vi "Can_Be_Package_Top_Level.vi"(8 "error in (no error)":errorcluster, 9 "AB_Source in":refnum<class "AB_Source.lvclass">, 11 "Build in":refnum<class "AB_Targetfile.lvclass">) -> (0 "error out":errorcluster, 2 "topLevel":bool, 3 "Build out":refnum<class "AB_Targetfile.lvclass">)   [LabVIEW 2020, in "AB_Targetfile.lvclass"]
uses:
  <vilib>/AppBuilder/AB_Classes/TargetFile/AB_Targetfile.lvclass
  <vilib>/AppBuilder/AB_Classes/Source/AB_Source.lvclass
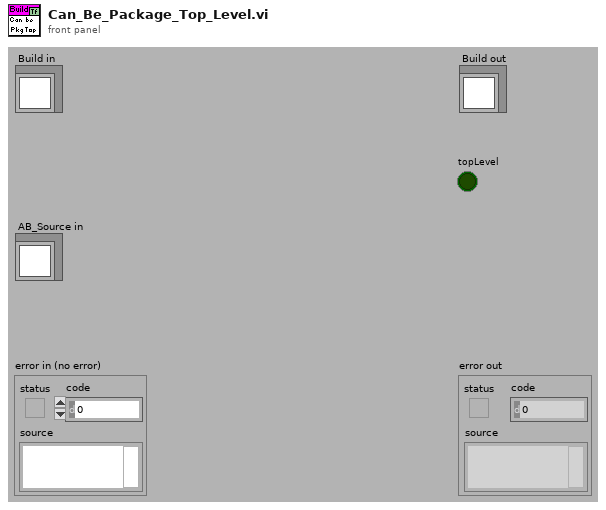
[diagram p1: front panel]
types:
  T1 = typedef "AB_Source.ctl" = cluster{"path":path, "itemID":string, "parentIndex":i32, "sourceInclusion":T2, "destinationIndex":i32, "properties":T3[], "newName":string, "lvfile":bool, "valid":bool, "eng_inBuild":bool, "eng_isNonVILink":bool, "Amalgamation":bool, "Amalgamation Piece":bool, "eng_delimitedName":string, "preventRename":bool}
  T2 = typedef "AB_Source_Inclusion.ctl" = enum16{"IncludeIfReferenced", "Include", "Exclude", "TopLevel"}
  T3 = typedef "AB_Source_Properties.ctl" = cluster{"sourcePropertyType":T4, "value":variant}
  T4 = typedef "AB_Source_Property_Type.ctl" = enum16{"Remove block diagram", "Remove front panel", "Password", "Window has title bar", "Show menu bar", "Show vertical scroll bar", "Show horizontal scroll bar", "Show toolbar", "Show Abort button", "Show fp when called", "Window behavior", "Allow user to close window", "Window run-time position", "Run when opened", "Allow debugging", "Auto error handling", "Generate guard code", "Use stack variables", "Expression folding", "Integer only", "Inline subVI"}
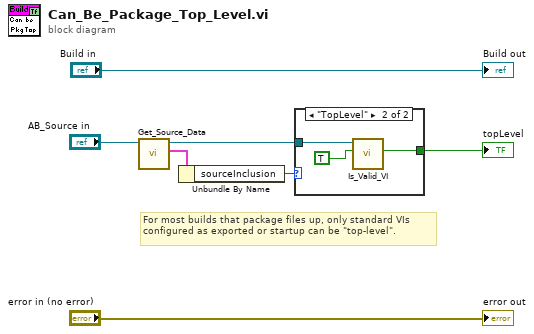
[diagram p0: block diagram]
diagram:
  # "For most builds that package files up, only standard VIs configured as exported or startup can be \"top-level\"."
  n1 = call <vilib>:"Get_Source_Data.vi"("Class in"="AB_Source in") -> ("data"=w5:T1, "Class out"=w3:refnum<class "AB_Source.lvclass">)  [unwired: 1 in, 8 out]
  n2 = Unbundle By Name(w5) -> ("sourceInclusion"=w2:T2)
  n3 = case shown="\"TopLevel\"" w2 {
    tunnel: w3 -> [_ w9]
    tunnel: [_ w8] -> w1
    frame Default {
    }
    frame "TopLevel" {
      n4 = call-dynamic "Is_Valid_VI.vi"("standardVI? (T)"=TRUE, "AB_Source in"=w9) -> ("VI"=w8:bool)  [unwired: 6 in, 3 out]
    }
  }
  "topLevel" <- w1
  "error out" <- "error in (no error)"
  "Build out" <- "Build in"
